vi "I2C Write.vi"(6 "Timeout ms (1000)":i32=1000, 7 "Slave Address (7-bit)":u8, 8 "Error In (No Error)":errorcluster, 9 "Keep Bus Busy":bool, 10 "Data to Write":u8[](array[numeric]), 11 "FPGA VI Reference In":T1) -> (0 "error out":errorcluster, 3 "FPGA VI Reference Out":T1)   [LabVIEW 2015]
uses:
  DSDB FPGA Ref.ctl
  <vilib>/rvi/errors/niLvFpgaAdjustHostInterfaceError.vi
  <vilib>/rvi/interface/nirviReadWriteControl/nirviReadWriteControl.xnode
  FPGA Bitfiles/Audio_FPGATarget_FPGAMain_3psOd07Wy8k.lvbitx
  FPGA Main.vi
  Sub VIs/Utilities/Start Boolean.ctl
  resource/NiAdept/NiAdept.dll
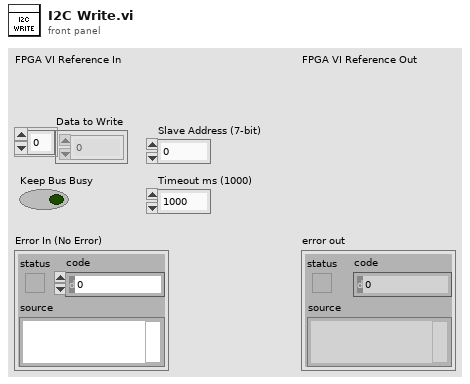
[diagram p1: front panel]
types:
  T1 = typedef "DSDB FPGA Ref.ctl" = refnum<k20>
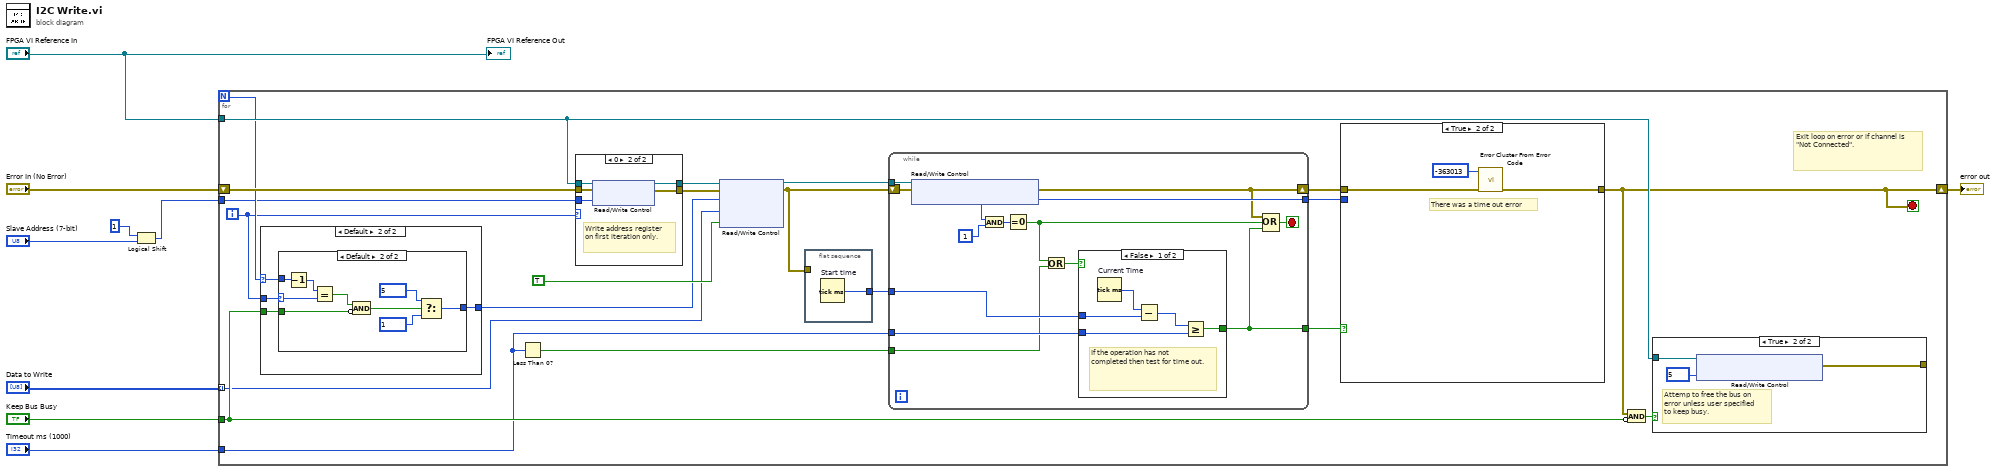
[diagram p0: block diagram]
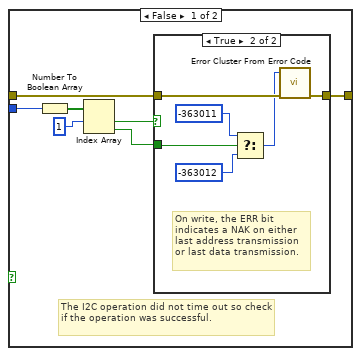
[diagram p2: hidden frame]
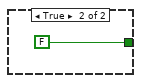
[diagram p6: hidden frame]
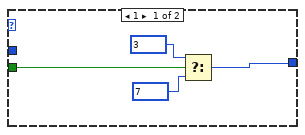
[diagram p7: hidden frame]
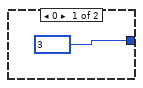
[diagram p8: hidden frame]
diagram:
  n1 = Logical Shift(y=i8 1, x="Slave Address (7-bit)") -> (x << y=w7:u8)
  n2 = for {
    N -> [w26]
    shift-right: [w10] -> w8
    shift-left: "Error In (No Error)" -> [w30]
    tunnel: "FPGA VI Reference In" -> [w29]
    tunnel: "Keep Bus Busy" -> [w23]
    tunnel: w7 -> [w25]
    tunnel: "Data to Write" -> [w22] mode=indexing
    tunnel: "Timeout ms (1000)" -> [w21]
    i -> [w24]
    stop <- w10 stop-if-true
    # "Exit loop on error or if channel is \"Not Connected\"."
    n3 = case shown="Default" w26 {
      selector: w26 -> [_ w83]
      tunnel: [w81 w84] -> w27
      tunnel: w24 -> [_ w85]
      tunnel: w23 -> [w79 w82]
      frame 1 {
        n4 = Select(t=u8 3 ("y"), s=w79, f=u8 7 ("y")) -> (s? t:f=w81:u8)
      }
      frame Default {
        n5 = case shown="Default" w85 {
          selector: w85 -> [_ w93]
          tunnel: [u8 3 ("y") w87] -> w84
          tunnel: w83 -> [_ w95]
          tunnel: w82 -> [_ w89]
          frame 0 {
          }
          frame Default {
            n6 = Decrement(x=w95) -> (x-1=w94:i32)
            n7 = Equal?(x=w94, y=w93) -> (x = y?=w90:bool)
            n8 = Compound Arithmetic op=AND(w90, invert w89) -> (w88:bool)
            n9 = Select(t=u8 5 ("y"), s=w88, f=u8 1 ("y")) -> (s? t:f=w87:u8)
          }
        }
      }
    }
    n10 = Less Than 0?(x=w21) -> (x < 0?=w20:bool)
    n11 = case shown="0" w24 {
      tunnel: [w53 w58] -> w16
      tunnel: [w52 w57] -> w15
      tunnel: w29 -> [w53 w56]
      tunnel: w30 -> [w52 w55]
      tunnel: w25 -> [_ w54]
      frame Default {
      }
      frame 0 {
        # "Write address register on first iteration only."
        n12 = xnode "Read/Write Control"("FPGA VI Reference In"=w56, "error in"=w55, "I2C.Address"=w54) -> ("FPGA VI Reference Out"=w58:T1, "error out"=w57:errorcluster)
      }
    }
    n13 = xnode "Read/Write Control"("FPGA VI Reference In"=w16, "error in"=w15, "I2C.Control"=w27, "I2C.DataOut"=w22, "I2C.GO"=TRUE ("I2C0.GO")) -> ("FPGA VI Reference Out"=w19:T1, "error out"=w11:errorcluster)
    n14 = flat-sequence {
      tunnel: [w31] -> w13
      tunnel: w11 -> [_]
      frame #0 {
        n15 = Tick Count (ms) "Start time"() -> (millisecond timer value=w31:u32)
      }
    }
    n16 = while {
      tunnel: w19 -> [w70]
      shift-right: [w65] -> w18
      shift-left: w11 -> [w71]
      tunnel: [w66] -> w17
      tunnel: w13 -> [w64]
      tunnel: [w63] -> w12
      tunnel: w21 -> [w62]
      tunnel: w20 -> [w59]
      stop <- w67 stop-if-true
      n17 = xnode "Read/Write Control"("FPGA VI Reference In"=w70, "error in"=w71) -> ("error out"=w65:errorcluster, "I2C.Status"=w66:u8)  [unwired: 1 out]
      n18 = And(x=w66, y=u8 1) -> (x .and. y?=w68:u8)
      n19 = Equal To 0?(x=w68) -> (x = 0?=w60:bool)
      n20 = Or(x=w60, y=w59) -> (x .or. y?=w61:bool)
      n21 = case shown="False" w61 {
        tunnel: w64 -> [w74 _]
        tunnel: [w73 FALSE] -> w63
        tunnel: w62 -> [w72 _]
        frame False {
          # "If the operation has not completed then test for time out."
          n22 = Tick Count (ms) "Current Time"() -> (millisecond timer value=w75:u32)
          n23 = Subtract(x=w75, y=w74) -> (x-y=w76:u32)
          n24 = Greater Or Equal?(x=w76, y=w72) -> (x >= y?=w73:bool)
        }
        frame True {
        }
      }
      n25 = Compound Arithmetic op=OR(w65, w60, w63) -> (w67:bool)
    }
    n26 = case shown="True" w12 {
      tunnel: w18 -> [w38 w47]
      tunnel: w17 -> [w37 _]
      tunnel: [w33 w46] -> w10
      frame False {
        # "The I2C operation did not time out so check if the operation was successful."
        n27 = Number To Boolean Array(number=w37) -> (Boolean array=w36:bool[])
        n28 = Index Array(array=w36, index #1=1 ("index")) -> (element #1=w35:bool, element #2=w32:bool)  [unwired: 1 in]
        n29 = case shown="True" w35 {
          tunnel: w38 -> [w39 w44]
          tunnel: [w39 w45] -> w33
          tunnel: w32 -> [_ w41]
          frame False {
          }
          frame True {
            # "On write, the ERR bit indicates a NAK on either last address transmission or last data transmission."
            n30 = Select(t=-363011, s=w41, f=-363012) -> (s? t:f=w42:i32)
            n31 = call <vilib>:"Error Cluster From Error Code.vi"("error in (no error)"=w44, "error code (0)"=w42) -> ("error out"=w45:errorcluster)  [unwired: 7 in]
          }
        }
      }
      frame True {
        # "There was a time out error"
        n32 = call <vilib>:"Error Cluster From Error Code.vi"("error in (no error)"=w47, "error code (0)"=-363013) -> ("error out"=w46:errorcluster)  [unwired: 7 in]
      }
    }
    n33 = Compound Arithmetic op=AND(w10, invert w23) -> (w14:bool)
    n34 = case shown="True" w14 {
      tunnel: w29 -> [_ w51]
      tunnel: [_ w49] -> _
      frame False {
      }
      frame True {
        # "Attemp to free the bus on error unless user specified to keep busy."
        n35 = xnode "Read/Write Control"("FPGA VI Reference In"=w51, "I2C.Control"=u8 5 ("I2C.C_0.CNTL")) -> ("error out"=w49:errorcluster)  [unwired: 1 in, 1 out]
      }
    }
  }
  "error out" <- w8
  "FPGA VI Reference Out" <- "FPGA VI Reference In"
